vi "AlliGator Find Object Python Function Information.vi"(8 "error in (no error)":errorcluster, 10 "Menu Item Tag":string, 11 "Object Refnum":refnum<vi>) -> (0 "error out":errorcluster, 1 "Found?":bool, 2 "Menu Item Tag (dup)":string, 3 "Python Function Info":T1)   [LabVIEW 2021, in "AlliGator Python Plugins.lvlib"]
doc: "Gets object's python function's information"
uses:
  AlliGator Python Plugins.lvlib
  AlliGator Python Function Information.ctl
  AlliGator Python Function Parameter Definition.ctl
  AlliGator Python Function Output Definition.ctl
  AlliGator Python Plugin Target Type.ctl
panel:
  # "see the AlliGator License on the block diagram (Ctrl+E or Window:Show Block Diagram)"
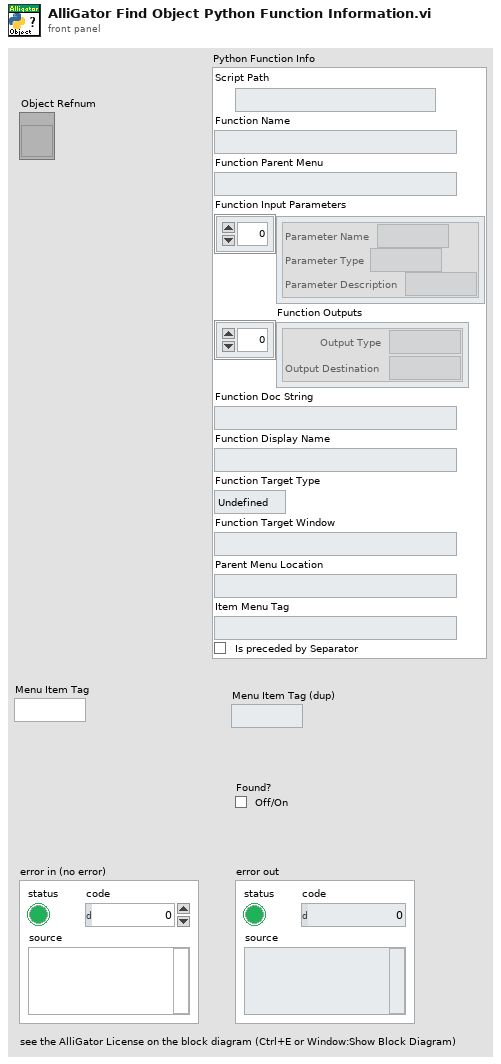
[diagram p1: front panel]
types:
  T1 = typedef "AlliGator Python Plugins.lvlib/AlliGator Python Function Information.ctl" = cluster{"Script Path":path, "Function Name":string, "Function Parent Menu":string, "Function Input Parameters":T2[], "Function Outputs":T3[], "Function Doc String":string, "Function Display Name":string, "Function Target Type":T4, "Function Target Window":string, "Parent Menu Location":string, "Item Menu Tag":string, "Is preceded by Separator":bool}
  T2 = typedef "AlliGator Python Plugins.lvlib/AlliGator Python Function Parameter Definition.ctl" = cluster{"Parameter Name":string, "Parameter Type":string, "Parameter Description":string}
  T3 = typedef "AlliGator Python Plugins.lvlib/AlliGator Python Function Output Definition.ctl" = cluster{"Output Type":string, "Output Destination":string}
  T4 = typedef "AlliGator Python Plugins.lvlib/AlliGator Python Plugin Target Type.ctl" = enum16{"Undefined", "Window Menu", "Object Menu"}
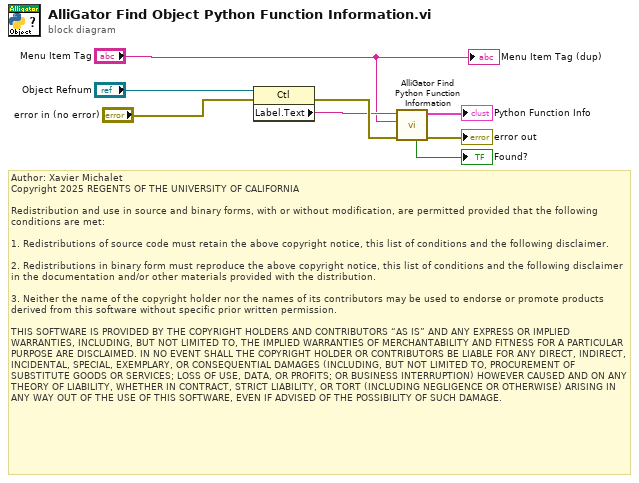
[diagram p0: block diagram]
diagram:
  # "Author: Xavier Michalet\nCopyright 2025 REGENTS OF THE UNIVERSITY OF CALIFORNIA\n\nRedistribution and use in source and binary forms, with or without modification, are permitted provided that the following conditions are met:\n\n1. Redistributions of source code must retain the above copyright notice, this list of conditions and the following disclaimer.\n\n2. Redistributions in binary form must reproduce the above copyright notice, this list of conditions and the following disclaimer in the documentation and/or other materials provided with the distribution.\n\n3. Neither the name of the copyright holder nor the names of its contributors may be used to endorse or promote products derived from this software without specific prior written permission.\n\nTHIS SOFTWARE IS PROVIDED BY THE COPYRIGHT HOLDERS AND CONTRIBUTORS “AS IS” AND ANY EXPRESS OR IMPLIED WARRANTIES, INCLUDING, BUT NOT LIMITED TO, THE IMPLIED WARRANTIES OF MERCHANTABILITY AND FITNESS FOR A PARTICULAR PURPOSE ARE DISCLAIMED. IN NO EVENT SHALL THE COPYRIGHT HOLDER OR CONTRIBUTORS BE LIABLE FOR ANY DIRECT, INDIRECT, INCIDENTAL, SPECIAL, EXEMPLARY, OR CONSEQUENTIAL DAMAGES (INCLUDING, BUT NOT LIMITED TO, PROCUREMENT OF SUBSTITUTE GOODS OR SERVICES; LOSS OF USE, DATA, OR PROFITS; OR BUSINESS INTERRUPTION) HOWEVER CAUSED AND ON ANY THEORY OF LIABILITY, WHETHER IN CONTRACT, STRICT LIABILITY, OR TORT (INCLUDING NEGLIGENCE OR OTHERWISE) ARISING IN ANY WAY OUT OF THE USE OF THIS SOFTWARE, EVEN IF ADVISED OF THE POSSIBILITY OF SUCH DAMAGE."
  n1 = property class="Ctl"(reference="Object Refnum", error in="error in (no error)") -> (error out=w4:errorcluster, "Label.Text"=w3:string)  [unwired: 1 out]
  n2 = call "AlliGator Find Python Function Information.vi"("error in (no error)"=w4, "Function Menu Item Tag"="Menu Item Tag", "Target"=w3) -> ("error out"=→"error out":errorcluster, "Python Function Info"=→"Python Function Info":T1, "Found?"=→"Found?":bool)  [unwired: 6 in]
  "Menu Item Tag (dup)" <- "Menu Item Tag"
